vi "Read Speed.vi"(8 "error in (no error)":errorcluster, 11 "Speed in":refnum<class "Speed.lvclass">) -> (0 "error out":errorcluster, 2 "Speed [u/s]":dbl, 3 "Speed out":refnum<class "Speed.lvclass">)   [LabVIEW 2013, in "HardwareCharacterization.lvlib" / "Speed.lvclass"]
uses:
  Speed.lvclass
  Speed.lvclass/Speed.ctl
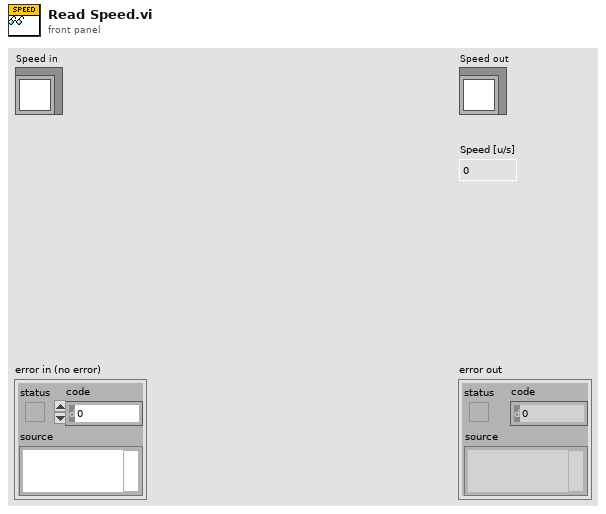
[diagram p1: front panel]
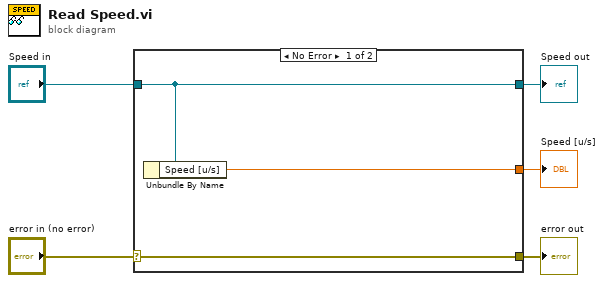
[diagram p0: block diagram]
diagram:
  n1 = case shown="No Error" "error in (no error)" {
    selector: "error in (no error)" -> [w8 w9]
    tunnel: [w8 w9] -> w4
    tunnel: [w7 w10] -> w2
    tunnel: "Speed in" -> [w7 w10]
    tunnel: [w6 _] -> w1
    frame No Error {
      n2 = Unbundle By Name(w7) -> ("Speed [u/s]"=w6:dbl)
    }
    frame Error {
    }
  }
  "error out" <- w4
  "Speed out" <- w2
  "Speed [u/s]" <- w1
